vi "Prompt_FileExists.vi"(0 "Project":u16(ring) items=["Proj_VaporTubes", "Proj_H2DT", "Proj_H2DT"], 1 "SubFolder":string="VAPORTUBE\\Temp Dependence", 2 "Meas. Description":string="Spectrometer_", 3 "Measurement number":i32) -> (4 "Measurement number 2":i32, 5 "Project 2":enum16{"H2TC", "VAPOR1"}(ring), 6 "SubFolder 2":string="VAPORTUBE\\Temp Dependence", 7 "Meas. Description 2":string="Spectrometer_", 8 "Overwrite":bool)   [LabVIEW 2018]
doc: "Displays a standard dialog box that prompts users to enter information, such as a user name and password.\n--------------------\n\nThis Express VI is configured as follows:\n\nMessage to Display to the User:\nThe inputs are: \nText Entry Box: Project\nText Entry Box: Measurement Description\nNumber: Measurement Number"
uses:
  <vilib>/Utility/file.llb/Read Delimited Spreadsheet (string).vi
panel:
  in  "Path":path=path "C:/Users/bowenm/Documents/ProjectIndex.csv"
  out "error out":errorcluster
  in  "error in (no error)":errorcluster
  out "String":string
  in  "Enable":bool=TRUE
  in  "Cancel":bool
  in  "OK2":bool
  in  "OK1":bool
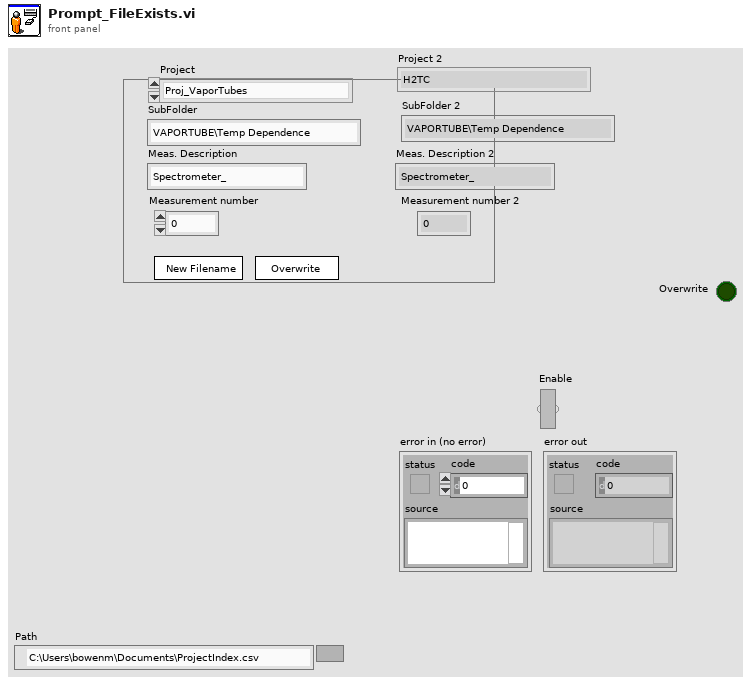
[diagram p1: front panel]
types:
  T1 = cluster{"Input Name":string, "Input Data Type":i32}[]
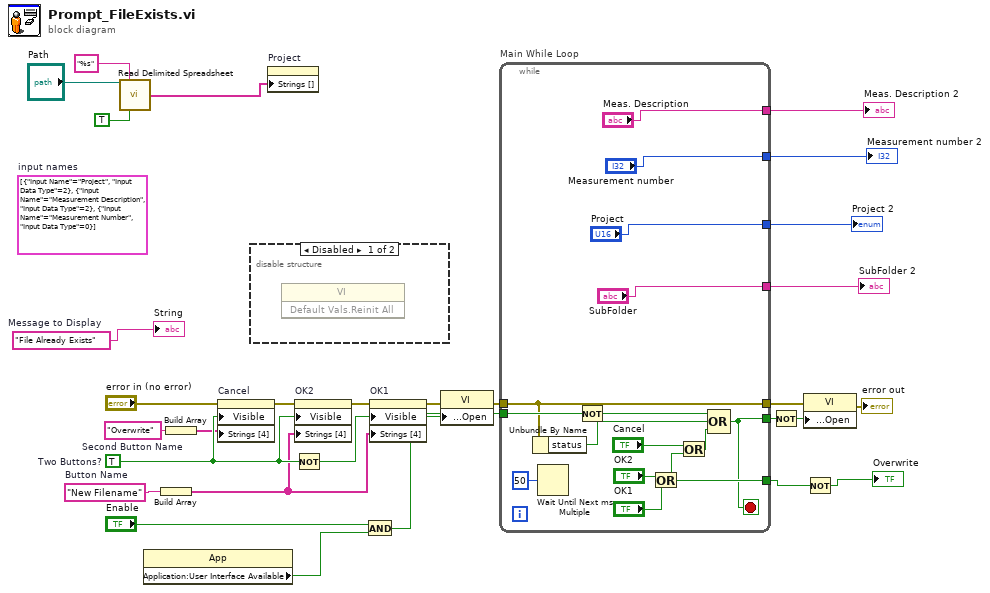
[diagram p0: block diagram]
diagram:
  (unwired) T1 [{"Input Name"="Project", "Input Data Type"=2}, {"Input Name"="Measurement Description", "Input Data Type"=2}, {"Input Name"="Measurement Number", "Input Data Type"=0}]  # input names
  w22 = "Overwrite"  # Second Button Name
  w20 = "New Filename"  # Button Name
  w11 = "File Already Exists"  # Message to Display
  w29 = TRUE  # Two Buttons?
  n1 = call-poly <vilib>:"Read Delimited Spreadsheet.vi"("file path (dialog if empty)"="Path", "format (%s)"="%s", "transpose? (F)"=TRUE) -> ("first row"=w1:string[])  [unwired: 7 in, 5 out]
  n2 = property class="App"() -> ("Application:User Interface Available"=w12:bool)  [unwired: 2 in, 2 out]
  n3 = Build Array(w20) -> (w21:string[])
  n4 = Build Array(w22) -> (w23:string[])
  n5 = property on="Cancel" class="Bool"(error in="error in (no error)", "Visible"=w29, "Strings [4]"=w23) -> (error out=w27:errorcluster)  [unwired: 1 in, 1 out]
  n6 = disable-structure shown="Disabled" {
    frame Disabled {
      n7 = invoke class="VI" method="Default Vals.Reinit All"() -> ()  [unwired: 3 in, 3 out]
    }
    frame Enabled {
    }
  }
  n8 = property on="Project" class="Ring (strict)"("Strings []"=w1) -> ()  [unwired: 2 in, 2 out]
  n9 = Not(x=w29) -> (.not. x?=w28:bool)
  n10 = property on="OK2" class="Bool"(error in=w27, "Visible"=w29, "Strings [4]"=w21) -> (error out=w26:errorcluster)  [unwired: 1 in, 1 out]
  n11 = And(x="Enable", y=w12) -> (x .and. y?=w13:bool)
  n12 = property on="OK1" class="Bool"(error in=w26, "Visible"=w28, "Strings [4]"=w21) -> (error out=w19:errorcluster)  [unwired: 1 in, 1 out]
  n13 = property class="VI"(error in=w19, "Front Panel Window:Open"=w13) -> (error out=w18:errorcluster)  [unwired: 1 in, 1 out]
  n14 = while "Main While Loop" {
    tunnel: [w41] -> w10
    tunnel: w13 -> [w39]
    tunnel: [w37] -> w24
    tunnel: w18 -> [w36]
    tunnel: [w36] -> w16
    tunnel: ["Meas. Description"] -> w8
    tunnel: ["Measurement number"] -> w7
    tunnel: ["Project"] -> w6
    tunnel: ["SubFolder"] -> w5
    stop <- w37 stop-if-true
    n15 = Unbundle By Name(w36) -> ("status"=w34:bool)
    n16 = Wait Until Next ms Multiple(millisecond multiple=u32 50) -> ()  [unwired: 1 out]
    n17 = Not(x=w39) -> (.not. x?=w38:bool)
    n18 = Or(x="OK2", y="OK1") -> (x .or. y?=w41:bool)
    n19 = Or(x="Cancel", y=w41) -> (x .or. y?=w35:bool)
    n20 = Compound Arithmetic op=OR(w38, w34, w35) -> (w37:bool)
  }
  "Meas. Description 2" <- w8
  "Measurement number 2" <- w7
  "SubFolder 2" <- w5
  "Project 2" <- w6
  n21 = Not(x=w24) -> (.not. x?=w25:bool)
  n22 = property class="VI"(error in=w16, "Front Panel Window:Open"=w25) -> (error out=→"error out":errorcluster)  [unwired: 1 in, 1 out]
  n23 = Not(x=w10) -> (.not. x?=→"Overwrite":bool)
  "String" <- w11
